vi "Time Setting Query.vi"(8 "error in (no error)":errorcluster, 11 "VISA resource name":refnum<visa-resource-name>) -> (0 "error out":errorcluster, 1 "Pulse Width (seconds)":dbl format="%^#_5g", 2 "Measurement Delay Time (seconds)":dbl format="%^#_5g", 3 "VISA resource name out":refnum<visa-resource-name>, 4 "Period (seconds)":dbl format="%^#_5g", 5 "Hold Time (seconds)":dbl format="%^#_5g")   [LabVIEW 2017, in "ADCMT 6240.lvlib"]
doc: "This VI returns time parameters which is read by \"SP?\" command.\n\n<B>Note:</B> Each parameters unit is a second."
uses:
  ADCMT 6240.lvlib
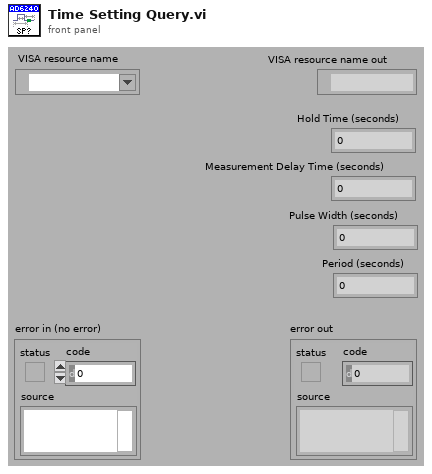
[diagram p1: front panel]
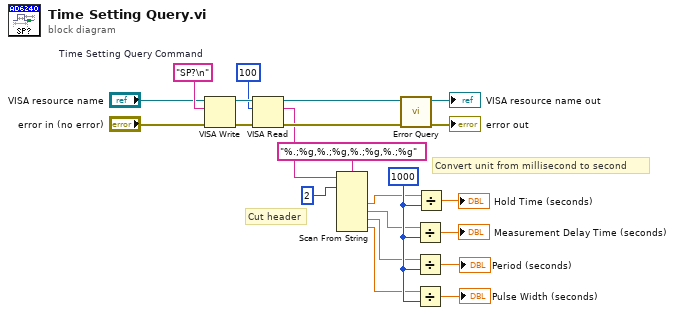
[diagram p0: block diagram]
diagram:
  w7 = 1000
  w17 = "SP?\n"  # Time Setting Query Command
  # "Convert unit from millisecond to second"
  # "Cut header"
  n1 = VISA Write(VISA resource name="VISA resource name", write buffer=w17, error in (no error)="error in (no error)") -> (VISA resource name out=w21:refnum<visa-resource-name>, error out=w22:errorcluster)  [unwired: 1 out]
  n2 = VISA Read(VISA resource name=w21, byte count=u32 100, error in (no error)=w22) -> (VISA resource name out=w14:refnum<visa-resource-name>, read buffer=w12:string, error out=w13:errorcluster)  [unwired: 1 out]
  n3 = Scan From String(format string="%.;%g,%.;%g,%.;%g,%.;%g", input string=w12, initial scan location=2) -> (output 1=w6:dbl, output 2=w3:dbl, output 3=w4:dbl, output 4=w5:dbl)  [unwired: 5 in, 3 out]
  n4 = call "Error Query.vi"("error in (no error)"=w13, "VISA resource name"=w14) -> ("error out"=→"error out":errorcluster, "VISA resource name out"=→"VISA resource name out":refnum<visa-resource-name>)  [unwired: 6 in, 2 out]
  n5 = Divide(x=w3, y=w7) -> (x/y=→"Measurement Delay Time (seconds)":dbl)
  n6 = Divide(x=w4, y=w7) -> (x/y=→"Period (seconds)":dbl)
  n7 = Divide(x=w5, y=w7) -> (x/y=→"Pulse Width (seconds)":dbl)
  n8 = Divide(x=w6, y=w7) -> (x/y=→"Hold Time (seconds)":dbl)
